vi "test_Update CD XML File_Error7001.vi"(8 "error in (no error)":errorcluster, 11 "TestCase in":refnum<class "LVLIBP CD XML Updater Unit Tests.lvclass">) -> (0 "error out":errorcluster, 3 "TestCase out":refnum<class "LVLIBP CD XML Updater Unit Tests.lvclass">)   [LabVIEW 2018, in "LVLIBP CD XML Updater Unit Tests.lvclass"]
uses:
  LVLIBP CD XML Updater Unit Tests.lvclass
  <vilib>/addons/_JKI Toolkits/VI Tester/TestCase.llb/TestCase.lvclass
  Utilities/.LVLIBP CD XML Updater/.LVLIBP CD XML Updater.lvlib
  Utilities/.LVLIBP CD XML Updater/Project XML Editor/Project XML Editor.lvclass
  FPGA Addon Test Class/FPGA Addon Test Class.lvclass
  C:/Program Files (x86)/National Instruments/LabVIEW 2018/vi.lib/addons/_JKI Toolkits/VI Tester/TestCase.llb/TestCase.lvclass
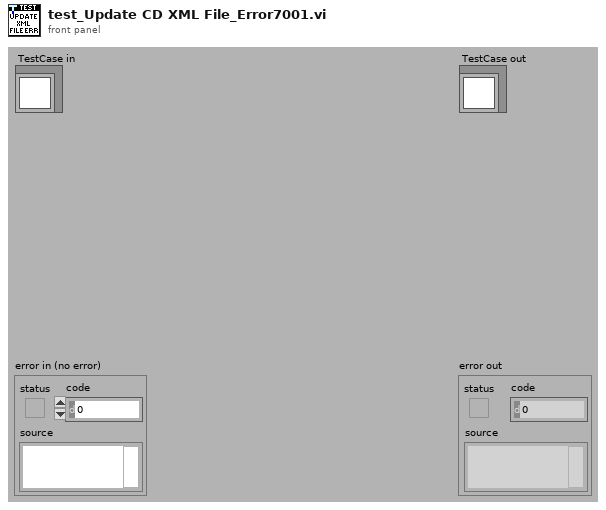
[diagram p1: front panel]
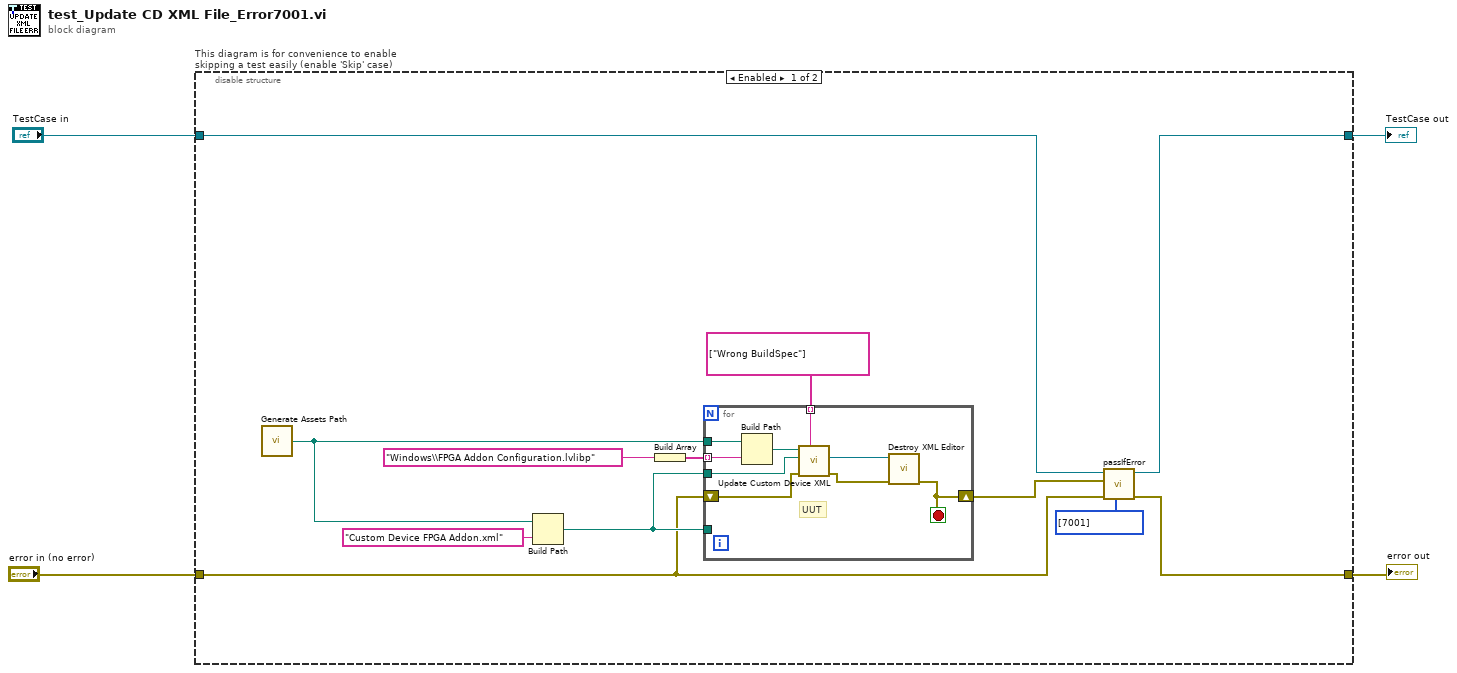
[diagram p0: block diagram]
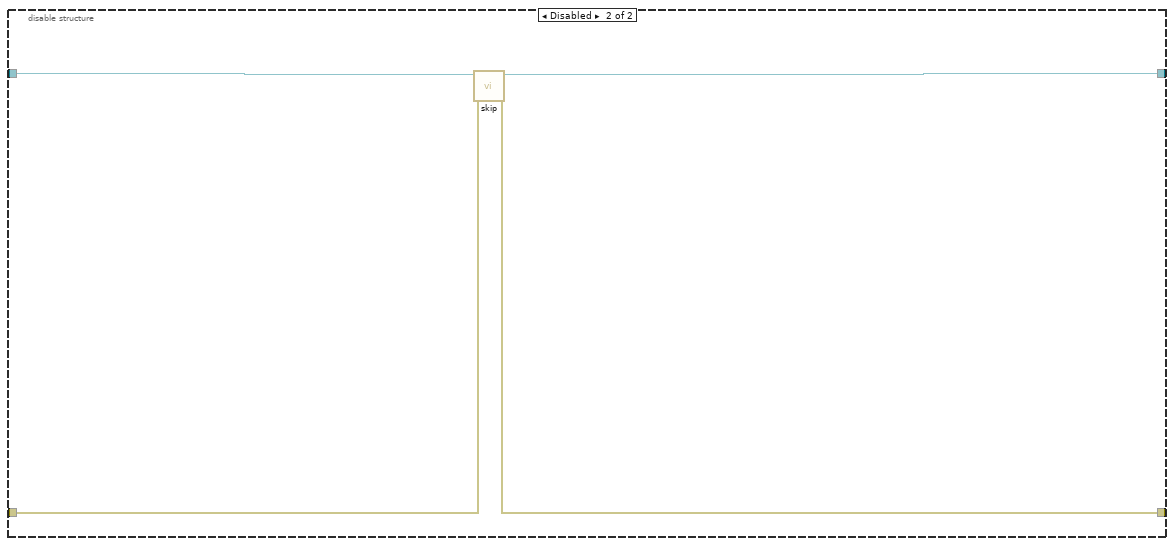
[diagram p2: hidden frame]
diagram:
  n1 = disable-structure "This diagram is for convenience to enable skipping a test easily (enable 'Skip' case)" shown="Enabled" {
    disable-tunnel: "TestCase in" -> [w10 w29]
    disable-tunnel: [w9 w27] -> w1
    disable-tunnel: [w8 w28] -> w3
    disable-tunnel: "error in (no error)" -> [w5 w26]
    frame Enabled {
      n2 = call "Generate Assets Path.vi"() -> ("Assets path"=w13:path)
      n3 = Build Path(base path=w13, name or relative path="Custom Device FPGA Addon.xml") -> (appended path=w11:path)
      n4 = Build Array("Windows\\FPGA Addon Configuration.lvlibp" ("name or relative path")) -> (w12:string[])
      n5 = for {
        tunnel: string[] ["Wrong BuildSpec"] -> [w25] mode=indexing
        tunnel: w11 -> [w24]
        shift-right: [w17] -> w6
        shift-left: w5 -> [w22]
        tunnel: w13 -> [w20]
        tunnel: w12 -> [w19] mode=indexing
        tunnel: w11 -> [_]
        stop <- w17 stop-if-true
        # "UUT"
        n6 = Build Path(base path=w20, name or relative path=w19) -> (appended path=w21:path)
        n7 = call "Update Custom Device XML.vi"("Build Spec Type"=w25, "error in (no error)"=w22, "CD XML/Project Path"=w24, "Packed Library Path"=w21) -> ("error out"=w23:errorcluster, "Project XML Editor out"=w18:refnum<class "Project XML Editor.lvclass">)  [unwired: 6 in]
        n8 = call "Destroy XML Editor.vi"("error in (no error)"=w23, "Project XML Editor in"=w18) -> ("error out"=w17:errorcluster)  [unwired: 9 in]
      }
      n9 = call-dynamic "passIfError.vi"("passing error codes (default = any error code)"=i32[] [7001], "error in (no error)"=w5, "error"=w6, "TestCase in"=w10) -> ("error out"=w8:errorcluster, "TestCase out"=w9:refnum<class "LVLIBP CD XML Updater Unit Tests.lvclass">)  [unwired: 6 in]
    }
    frame Disabled {
      # "skip test result while test is under development"
      n10 = call <vilib>:"skip.vi"("error in (no error)"=w26, "TestCase in"=w29) -> ("error out"=w28:errorcluster, "TestCase out"=w27:refnum<class "LVLIBP CD XML Updater Unit Tests.lvclass">)  [unwired: 8 in]
    }
  }
  "error out" <- w3
  "TestCase out" <- w1
